vi "score_samples.vi"(8 "error in (no error)":errorcluster caption="entrée d'erreur (pas d'erreur)", 11 "Mixture.lvclass 2":refnum<class "Mixture.lvclass">) -> (0 "error out":errorcluster caption="sortie d'erreur", 2 "scores":dbl[](array[numeric]), 3 "Mixture.lvclass":refnum<class "Mixture.lvclass">)   [LabVIEW 2020, in "Mixture.lvclass"]
doc: "Compute the weighted log probabilities for each sample."
uses:
  Mixture.lvclass
  C:/Users/cipop/TDF Dropbox/2_Technologies de France/1 - Services et Etudes/PLAIY/2 - DEV/PLAIYLAB/code/Model/Model.lvclass
  C:/Users/cipop/TDF Dropbox/2_Technologies de France/1 - Services et Etudes/PLAIY/2 - DEV/PLAIYLAB/code/Python/Python.lvclass
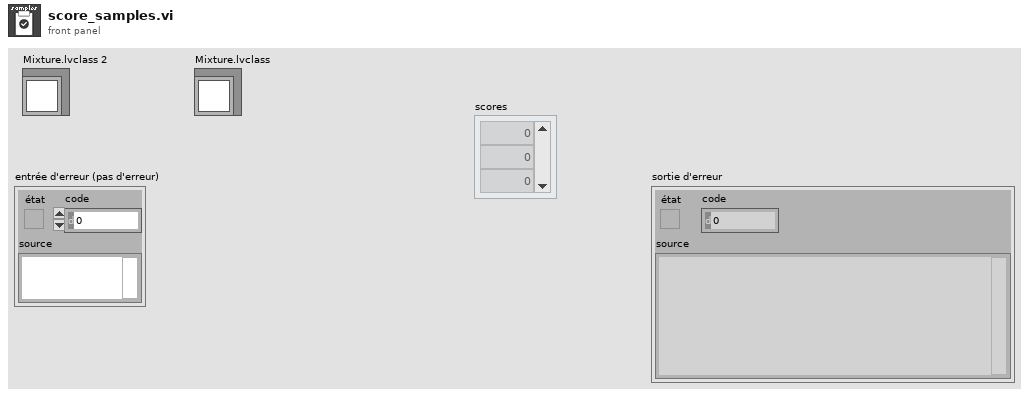
[diagram p1: front panel]
types:
  T1 = typedef "data.ctl" = cluster{"name":string, "X":dbl[][]}
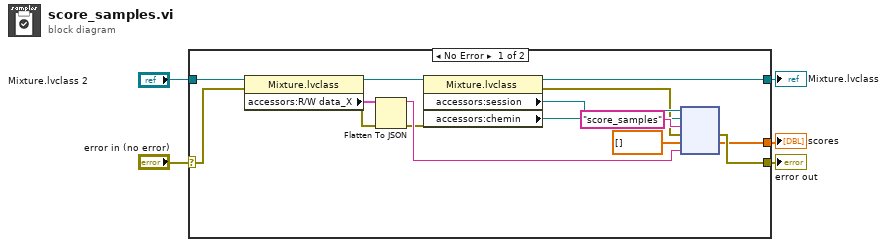
[diagram p0: block diagram]
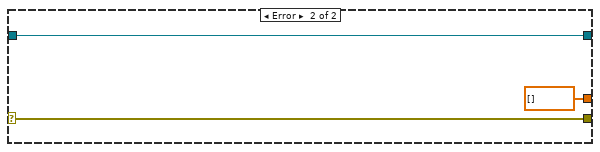
[diagram p2: hidden frame]
diagram:
  n1 = case shown="No Error" "error in (no error)" {
    selector: "error in (no error)" -> [w13 w23]
    tunnel: [w19 w23] -> w4
    tunnel: [w18 w22] -> w2
    tunnel: "Mixture.lvclass 2" -> [w12 w22]
    tunnel: [w6 dbl[] [] ("Numeric")] -> w1
    frame No Error {
      n2 = property class="Mixture.lvclass"(reference=w12, error in=w13) -> (reference out=w14:refnum<class "Mixture.lvclass">, error out=w9:errorcluster, "accessors:R/W data_X"=w11:T1)
      n3 = Flatten To JSON(anything=w11, error in (no error)=w9) -> (JSON string=w10:string, 11:w8:errorcluster)  [unwired: 1 in]
      n4 = property class="Mixture.lvclass"(reference=w14, error in=w8) -> (reference out=w18:refnum<class "Mixture.lvclass">, error out=w15:errorcluster, "accessors:session"=w17:refnum<k35>, "accessors:chemin"=w16:path)
      n5 = node(w17, w16, "score_samples" ("nom de la fonction"), w15, dbl[] [] ("Numeric"), w10) -> (w19:errorcluster, w6:dbl[])  [unwired: 1 in, 3 out]
    }
    frame Error {
    }
  }
  "scores" <- w1
  "error out" <- w4
  "Mixture.lvclass" <- w2
